vi "Stop.vi"(0 "Universal Robot.lvclass in":refnum<class "Universal Robot.lvclass">, 5 "error in (no error)":errorcluster) -> (14 "Universal Robot.lvclass out":refnum<class "Universal Robot.lvclass">, 19 "error out":errorcluster)   [LabVIEW 2019, in "Universal Robot.lvclass"]
uses:
  Universal Robot.lvclass
  ProgramControlEvent.ctl
  Universal Robot.lvclass/Universal Robot.ctl
  Client Interfaces/Dashboard Server/Dashboard Server.lvclass
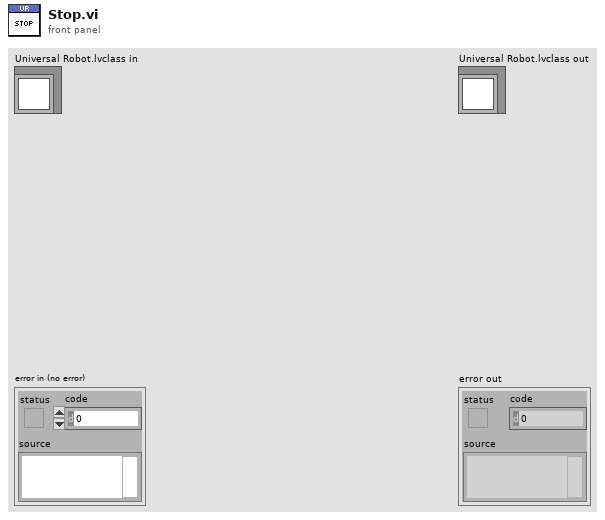
[diagram p1: front panel]
types:
  T1 = typedef "Universal Robot.lvclass/ProgramControlEvent.ctl" = enum16{"Stop", "Pause", "Resume"}
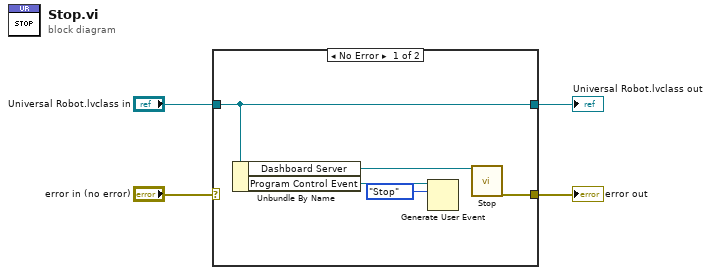
[diagram p0: block diagram]
diagram:
  n1 = case shown="No Error" "error in (no error)" {
    selector: "error in (no error)" -> [_ w11]
    tunnel: [w8 w11] -> w3
    tunnel: "Universal Robot.lvclass in" -> [w9 w10]
    tunnel: [w9 w10] -> w1
    frame No Error {
      n2 = Unbundle By Name(w9) -> ("Dashboard Server"=w7:refnum<class "Dashboard Server.lvclass">, "Program Control Event"=w6:refnum<user-event>)
      n3 = Generate User Event(user event=w6, event data cluster=ProgramControlEvent."Stop" ("event data")) -> ()  [unwired: 2 in, 2 out]
      n4 = call-dynamic "Stop.vi"("DashboardServer in"=w7) -> ("error out"=w8:errorcluster)  [unwired: 17 in, 1 out]
    }
    frame Error {
    }
  }
  "error out" <- w3
  "Universal Robot.lvclass out" <- w1
